vi "滚轮操作.vi"(8 "error in (no error)":errorcluster caption="错误输入（无错误）", 11 "程序响应 输入":refnum<class "程序响应.lvclass">) -> (0 "error out":errorcluster caption="错误输出", 3 "程序响应 输出":refnum<class "程序响应.lvclass">)   [LabVIEW 2018, in "程序响应.lvlib" / "程序响应.lvclass"]
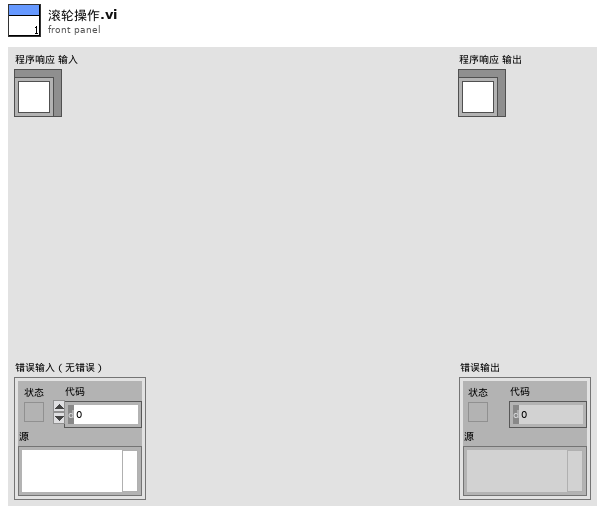
[diagram p1: front panel]
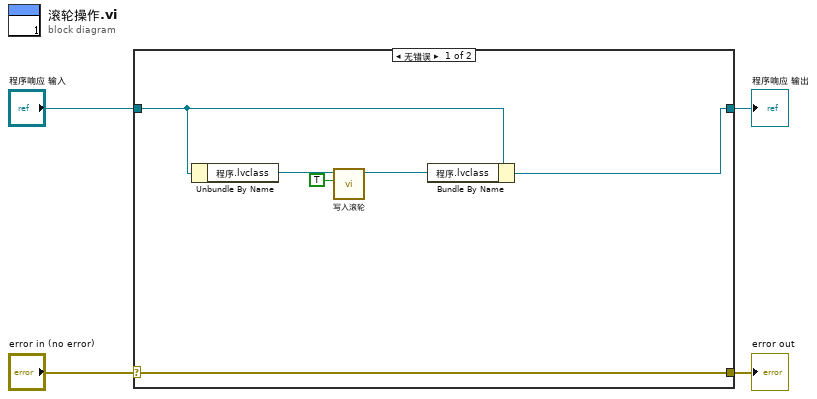
[diagram p0: block diagram]
diagram:
  n1 = case shown="无错误" "error in (no error)" {
    selector: "error in (no error)" -> [w10 w12]
    tunnel: [w10 w12] -> w3
    tunnel: [w5 w11] -> w1
    tunnel: "程序响应 输入" -> [w6 w11]
    frame No Error {
      n2 = Unbundle By Name(w6) -> ("程序.lvclass"=w9:refnum<class "程序.lvclass">)
      n3 = call-dynamic "写入滚轮.vi"("滚轮"=TRUE, "程序输入"=w9) -> ("程序输出"=w7:refnum<class "程序.lvclass">)  [unwired: 8 in, 1 out]
      n4 = Bundle By Name(cluster=w6, "程序.lvclass"=w7) -> (w5:refnum<class "程序响应.lvclass">)
    }
    frame Error {
    }
  }
  "error out" <- w3
  "程序响应 输出" <- w1
